vi "Day03-01_상태 머신 구조.vi"() -> ()   [LabVIEW 2021]
panel:
  out "경과 시간(ms)":u32
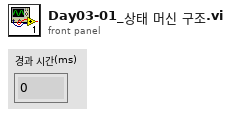
[diagram p1: front panel]
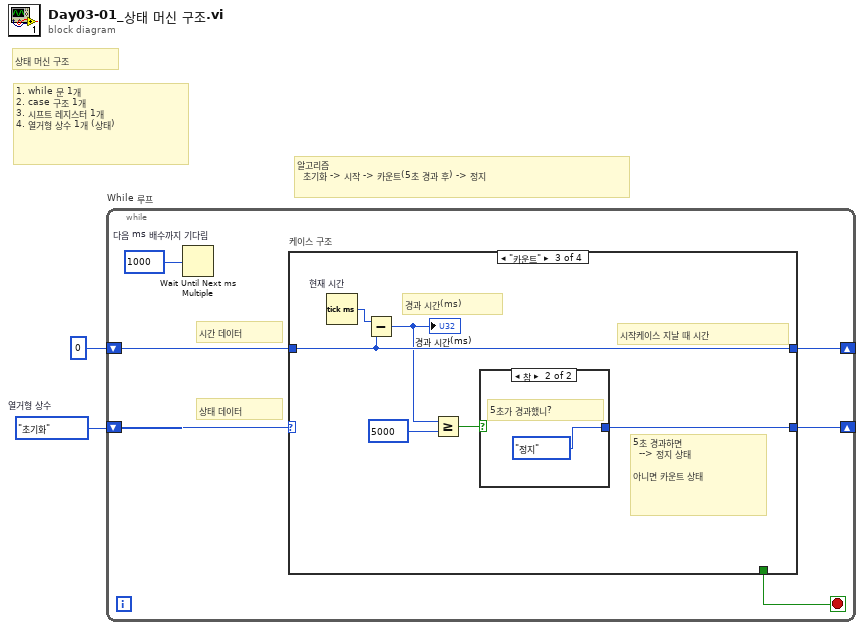
[diagram p0: block diagram]
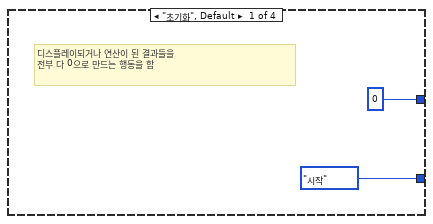
[diagram p2: hidden frame]
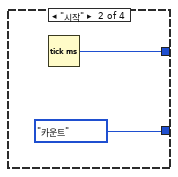
[diagram p3: hidden frame]
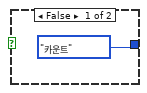
[diagram p4: hidden frame]
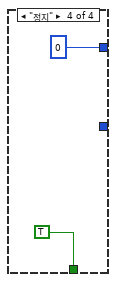
[diagram p5: hidden frame]
diagram:
  w2 = enum16{"초기화", "시작", "카운트", "정지"}."초기화"  # 열거형 상수
  # "상태 머신 구조"
  # "알고리즘\n  초기화 -> 시작 -> 카운트(5초 경과 후) -> 정지"
  # "1. while 문 1개\n2. case 구조 1개\n3. 시프트 레지스터 1개\n4. 열거형 상수 1개 (상태)"
  n1 = while "While 루프" {
    shift-right: [w7] -> _
    shift-left: w2 -> [w8]
    shift-right: [w5] -> _
    shift-left: 0 -> [w6]
    stop <- w4 stop-if-true
    # "상태 데이터"
    # "시간 데이터"
    n2 = Wait Until Next ms Multiple "다음 ms 배수까지 기다림"(millisecond multiple=u32 1000 ("ms 배수")) -> ()  [unwired: 1 out]
    n3 = case "케이스 구조" shown="\"카운트\"" w8 {
      tunnel: [enum16{"초기화", "시작", "카운트", "정지"}."시작" enum16{"초기화", "시작", "카운트", "정지"}."카운트" w14 _] -> w7
      tunnel: w6 -> [_ _ w17 _]
      tunnel: [0 w11 w17 0] -> w5
      tunnel: [_ _ _ TRUE] -> w4
      frame "초기화", Default {
        # "디스플레이되거나 연산이 된 결과들을\n전부 다 0으로 만드는 행동을 함"
      }
      frame "시작" {
        n4 = Tick Count (ms)() -> (millisecond timer value=w11:u32)
      }
      frame "카운트" {
        # "5초 경과하면\n  --> 정지 상태\n\n아니면 카운트 상태"
        # "경과 시간(ms)"
        # "시작케이스 지날 때 시간"
        n5 = Tick Count (ms) "현재 시간"() -> (millisecond timer value=w18:u32)
        n6 = Subtract(x=w18, y=w17) -> (x-y=w16:u32)
        "경과 시간(ms)" <- w16
        n7 = Greater Or Equal?(x=w16, y=u32 5000) -> (x >= y?=w13:bool)
        n8 = case shown="참" w13 {
          tunnel: [enum16{"초기화", "시작", "카운트", "정지"}."카운트" enum16{"초기화", "시작", "카운트", "정지"}."정지"] -> w14
          frame False {
          }
          frame True {
            # "5초가 경과했니?"
          }
        }
      }
      frame "정지" {
      }
    }
  }
